vi "Set Node Names.vi"(6 "Node ID":u32, 8 "Node":string, 9 "Cluster":string, 10 "System":string, 11 "Module in":refnum<class "Module.lvclass">) -> (3 "Module out":refnum<class "Module.lvclass">)   [LabVIEW 2020, in "Volatus.lvlib" / "Module.lvclass"]
uses:
  Module.lvclass
  Module.lvclass/Module.ctl
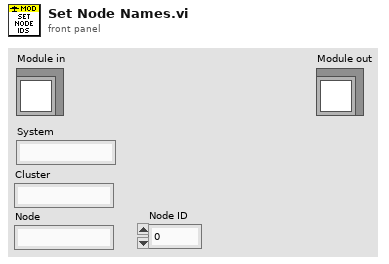
[diagram p1: front panel]
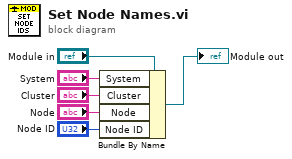
[diagram p0: block diagram]
diagram:
  n1 = Bundle By Name(cluster="Module in", "System"="System", "Cluster"="Cluster", "Node"="Node", "Node ID"="Node ID") -> (→"Module out":refnum<class "Module.lvclass">)
